vi "Filter Unexpired Paths.vi"(0 "Path Group in":refnum<class "Path Group.lvclass">, 11 "error in (no error)":errorcluster) -> (4 "Path Group out":refnum<class "Path Group.lvclass">, 6 "Expired Path Count":i32, 10 "Paths Filtered out":refnum<class "Path.lvclass">[](array[class]), 15 "error out":errorcluster)   [LabVIEW 2023, in "RFCalAndFixtureCharact.Common.lvlib" / "Path Group.lvclass"]
uses:
  Path Group.lvclass
  Path/Path.lvclass
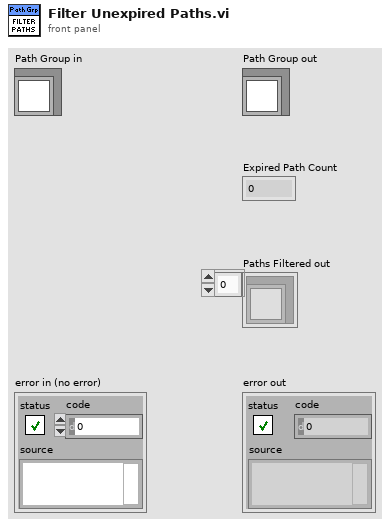
[diagram p1: front panel]
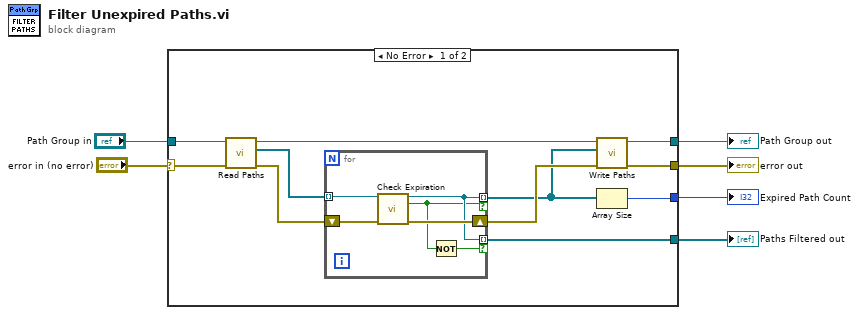
[diagram p0: block diagram]
diagram:
  n1 = case shown="No Error" "error in (no error)" {
    selector: "error in (no error)" -> [w17 w25]
    tunnel: [w12 w25] -> w5
    tunnel: [w10 w24] -> w3
    tunnel: "Path Group in" -> [w16 w24]
    tunnel: [w8 _] -> w2
    tunnel: [w7 _] -> w1
    frame No Error {
      n2 = call-dynamic "Read Paths.vi"("error in (no error)"=w17, "Cable Path Group in"=w16) -> ("error out"=w13:errorcluster, "Paths"=w15:refnum<class "Path.lvclass">[], "Cable Path Group out"=w11:refnum<class "Path Group.lvclass">)  [unwired: 7 in]
      n3 = for {
        tunnel: w15 -> [w21] mode=indexing
        shift-right: [w22] -> w14
        shift-left: w13 -> [w23]
        tunnel: [w20] -> w9 mode=indexing if=w19
        tunnel: [w20] -> w7 mode=indexing if=w18
        n4 = call "Check Expiration.vi"("Path in"=w21, "error in (no error)"=w23) -> ("Path out"=w20:refnum<class "Path.lvclass">, "Expired?"=w19:bool, "error out"=w22:errorcluster)  [unwired: 11 in]
        n5 = Not(x=w19) -> (.not. x?=w18:bool)
      }
      n6 = call-dynamic "Write Paths.vi"("error in (no error)"=w14, "Paths"=w9, "Cable Path Group in"=w11) -> ("error out"=w12:errorcluster, "Cable Path Group out"=w10:refnum<class "Path Group.lvclass">)  [unwired: 7 in]
      n7 = Array Size(array=w9) -> (size(s)=w8:i32)
    }
    frame Error {
    }
  }
  "error out" <- w5
  "Path Group out" <- w3
  "Expired Path Count" <- w2
  "Paths Filtered out" <- w1
